vi "Write Laser.vi"(7 "analisysMeth":cluster{"Red":T1, "Blue":T1, "Green":T1}, 8 "error in":errorcluster, 9 "Wavelength":cluster{"Red":dbl, "Blue":dbl, "Green":dbl}, 10 "Laser":T2=enum."Blue", 11 "CRDS Cell in":refnum<class "CRDS Cell.lvclass">=refnum) -> (0 "error out":errorcluster, 3 "CRDS Cell out":refnum<class "CRDS Cell.lvclass">)   [LabVIEW 2012]
uses:
  CRDS Cell.lvclass
  PAS_CRDS new/CRDS/Controls/las_lambda.ctl
  Instruments/cPAS/Interface/CRDS/Controls/analys_meth.ctl
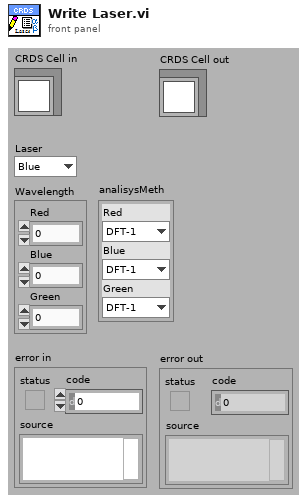
[diagram p1: front panel]
types:
  T1 = typedef "analys_meth.ctl" = enum16{"DFT-1", "DFT-5", "LRS"}
  T2 = typedef "las_lambda.ctl" = enum16{"Red", "Blue", "Green"}
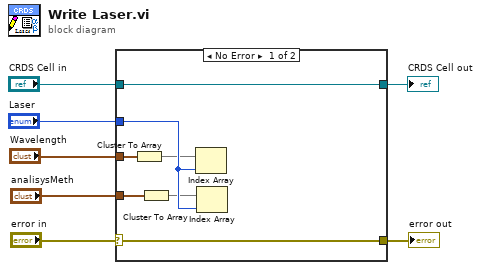
[diagram p0: block diagram]
diagram:
  n1 = case shown="No Error" "error in" {
    selector: "error in" -> [w14 w15]
    tunnel: [w14 w15] -> w6
    tunnel: [w8 w16] -> w4
    tunnel: "CRDS Cell in" -> [w8 w16]
    tunnel: "Laser" -> [w13 _]
    tunnel: "Wavelength" -> [w12 _]
    tunnel: "analisysMeth" -> [w11 _]
    frame No Error {
      n2 = Cluster To Array(cluster=w12) -> (array=w10:dbl[])
      n3 = Cluster To Array(cluster=w11) -> (array=w9:T1[])
      n4 = Index Array(array=w10, index=w13) -> ()  [unwired: 1 out]
      n5 = Index Array(array=w9, index=w13) -> ()  [unwired: 1 out]
    }
    frame Error {
    }
  }
  "error out" <- w6
  "CRDS Cell out" <- w4
